vi "Write CCD Config.vi"(8 "error in (no error)":errorcluster, 10 "CCD Config":T1={"Exposure Time"=1.0, "Pre-amp gain"=0, "Readout Rate"=0, "EM Mode"=1, "EM Gain"=2, "Binning"=1, "Initial Line"=1, "Initial Cloumn"=1, "Final Line"=1024, "Final Column"=1024, "Kinetic Series Length"=1, "Shutter Mode"=2, "Cooler ON/OFF"=0, "Temperature"=20, "Cubes"=1, "Trigger"=0} {"Trigger" items=["Internal", "External", "-", "-", "-", "-", "External Start"]; "Temperature" min=0 max=0; "Cooler ON/OFF" items=["Cooler OFF", "Cooler ON"]; "Shutter Mode" items=["Fully Auto", "OPEN", "CLOSED"]; "EM Mode" items=["Electron Multiplying", "Conventional"]; "Readout Rate" items=["1 MHz", "10 MHz", "20 MHz", "30 MHz"]; "Pre-amp gain" items=["Gain 1", "Gain 2"]}, 11 "JSON reader in":refnum<class "JSON reader.lvclass">) -> (0 "error out":errorcluster, 3 "JSON reader out":refnum<class "JSON reader.lvclass">)   [LabVIEW 2018, in "JSON reader.lvclass"]
uses:
  JSON reader.lvclass
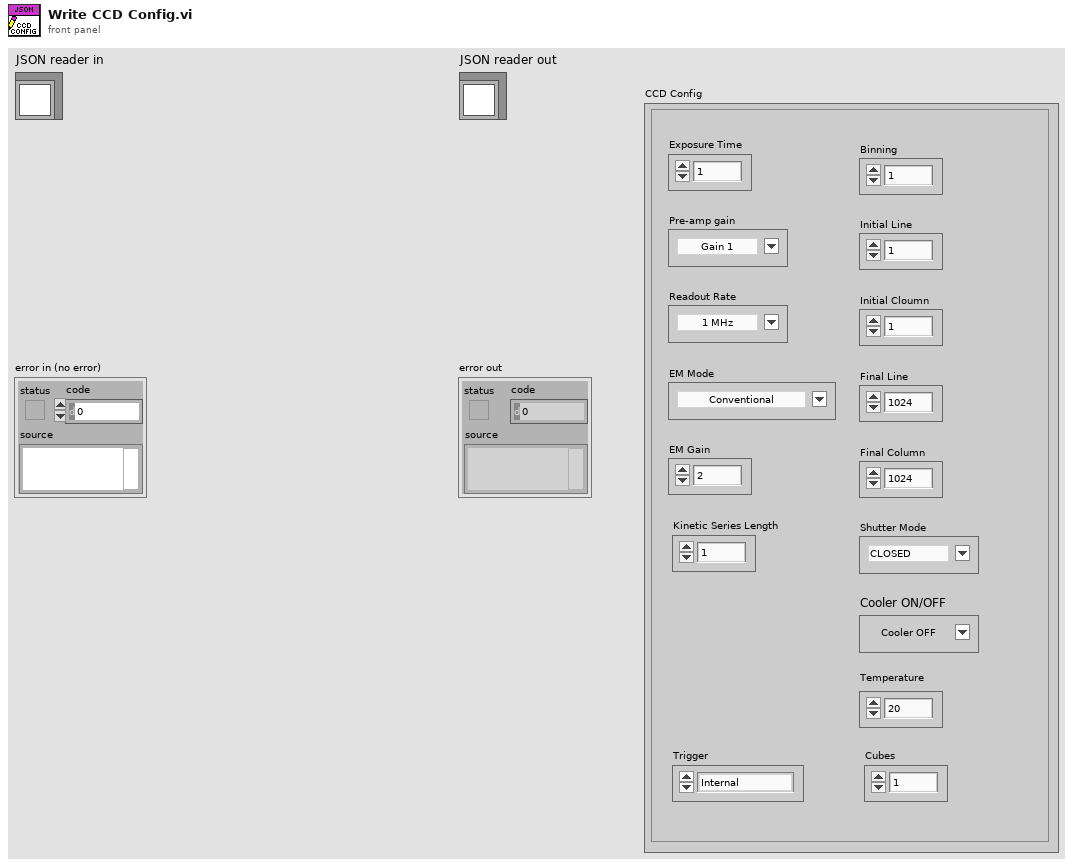
[diagram p1: front panel]
types:
  T1 = cluster{"Exposure Time":sgl, "Pre-amp gain":u8, "Readout Rate":u8, "EM Mode":u8, "EM Gain":u16, "Binning":u16, "Initial Line":u16, "Initial Cloumn":u16, "Final Line":u16, "Final Column":u16, "Kinetic Series Length":u32, "Shutter Mode":u8, "Cooler ON/OFF":u16, "Temperature":i8, "Cubes":u32, "Trigger":u16}
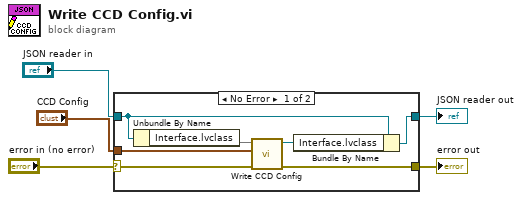
[diagram p0: block diagram]
diagram:
  n1 = case shown="No Error" "error in (no error)" {
    selector: "error in (no error)" -> [w8 w13]
    tunnel: [w7 w13] -> w4
    tunnel: [w12 w14] -> w2
    tunnel: "JSON reader in" -> [w11 w14]
    tunnel: "CCD Config" -> [w6 _]
    frame No Error {
      n2 = Unbundle By Name(w11) -> ("Interface.lvclass"=w9)
      n3 = call "Write CCD Config.vi"("error in (no error)"=w8, "CCD Config"=w6, "JSON reader in"=w9) -> ("error out"=w7:errorcluster, "JSON reader out"=w10:refnum<class "JSON reader.lvclass">)  [unwired: 7 in]
      n4 = Bundle By Name(cluster=w11, "Interface.lvclass"=w10) -> (w12:refnum<class "JSON reader.lvclass">)
    }
    frame Error {
    }
  }
  "error out" <- w4
  "JSON reader out" <- w2
